vi "04 - Run lifecycle.vi"   [LabVIEW 2020]
uses:
  client/client.lvlib
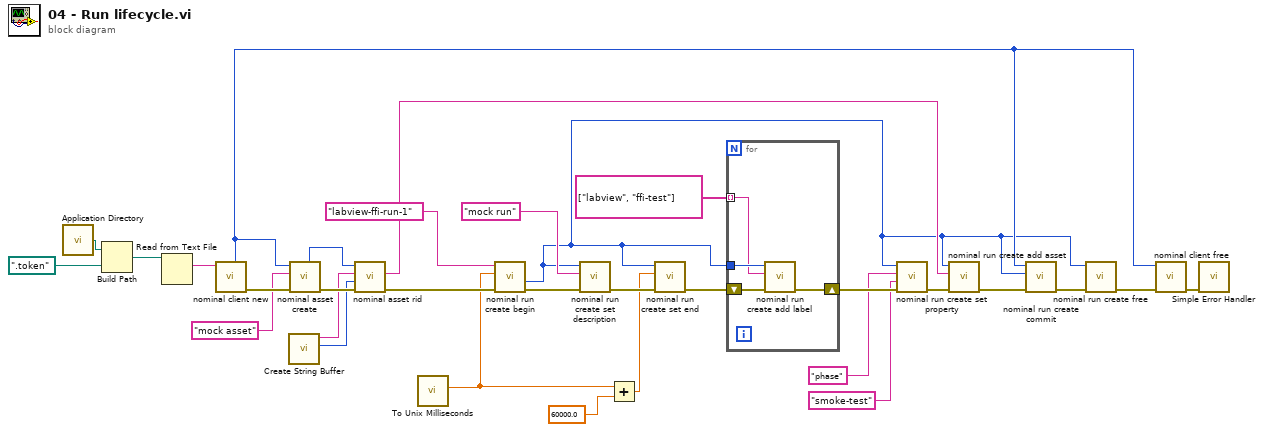
[diagram p0: block diagram]
diagram:
  n1 = call <vilib>:"Application Directory.vi"() -> ("Application Directory"=w30:path)
  n2 = Build Path(base path=w30, name or relative path=path ".token") -> (appended path=w28:path)
  n3 = Read from Text File(file (use dialog)=w28) -> (text=w27:string)  [unwired: 3 in, 3 out]
  n4 = call "nominal client new.vi"("token"=w27) -> ("error out"=w26:errorcluster, "out_client out"=w8:i32)  [unwired: 8 in, 1 out]
  n5 = call "Create String Buffer.vi"() -> ("dub Buffer Size"=w2:i32, "String Buffer"=w3:string)  [unwired: 9 in, 1 out]
  n6 = call "nominal asset create.vi"("error in (no error)"=w26, "name"="mock asset", "client"=w8) -> ("error out"=w24:errorcluster, "out_asset out"=w25:i32)  [unwired: 6 in, 1 out]
  n7 = call "nominal asset rid.vi"("error in (no error)"=w24, "cap"=w2, "buf"=w3, "asset"=w25) -> ("error out"=w21:errorcluster, "buf out"=w10:string)  [unwired: 4 in, 2 out]
  n8 = call "To Unix Milliseconds.vi"() -> ("Unix Milliseconds"=w1:dbl)  [unwired: 11 in]
  n9 = call "nominal run create begin.vi"("error in (no error)"=w21, "start_ms"=w1, "name"="labview-ffi-run-1") -> ("error out"=w20:errorcluster, "out_staging out"=w6:i32)  [unwired: 6 in, 1 out]
  n10 = call "nominal run create set description.vi"("error in (no error)"=w20, "description"="mock run" ("name"), "staging"=w6) -> ("error out"=w18:errorcluster)  [unwired: 7 in, 1 out]
  n11 = Add(x=w1, y=60000.0) -> (x+y=w16:dbl)
  n12 = call "nominal run create set end.vi"("error in (no error)"=w18, "end_ms"=w16, "staging"=w6) -> ("error out"=w15:errorcluster)  [unwired: 7 in, 1 out]
  n13 = for {
    tunnel: w6 -> [w35]
    tunnel: string[] ["labview", "ffi-test"] ("name") -> [w33] mode=indexing
    shift-right: [w32] -> w13
    shift-left: w15 -> [w34]
    n14 = call "nominal run create add label.vi"("error in (no error)"=w34, "label"=w33, "staging"=w35) -> ("error out"=w32:errorcluster)  [unwired: 7 in, 1 out]
  }
  n15 = call "nominal run create set property.vi"("error in (no error)"=w13, "value"="smoke-test" ("name"), "key"="phase" ("name"), "staging"=w6) -> ("error out"=w9:errorcluster)  [unwired: 6 in, 1 out]
  n16 = call "nominal run create add asset.vi"("error in (no error)"=w9, "asset_rid"=w10, "staging"=w6) -> ("error out"=w7:errorcluster)  [unwired: 7 in, 1 out]
  n17 = call "nominal run create commit.vi"("error in (no error)"=w7, "staging"=w6, "client"=w8) -> ("error out"=w5:errorcluster)  [unwired: 6 in, 2 out]
  n18 = call "nominal run create free.vi"("error in (no error)"=w5, "staging"=w6) -> ("error out"=w4:errorcluster)  [unwired: 8 in, 1 out]
  n19 = call "nominal client free.vi"("error in (no error)"=w4, "client"=w8) -> ("error out"=w31:errorcluster)  [unwired: 8 in, 1 out]
  n20 = call <vilib>:"Simple Error Handler.vi"("error in (no error)"=w31) -> ()  [unwired: 4 in, 5 out]
